vi "Send Throttle Signal.vi"(8 "error in (no error)":errorcluster, 9 "Requested Torque (Nm)":dbl format="%#_13g", 10 "CAN Offset":u32=160 format="%x", 11 "interface object in":refnum<k20>) -> (0 "error out":errorcluster, 3 "interface object out":refnum<k20>)   [LabVIEW 2014]
uses:
  <vilib>/RioEmbeddedCAN/RioEmbeddedCAN.llb/CANFrameControl.ctl
panel:
  in  "Direction":u8
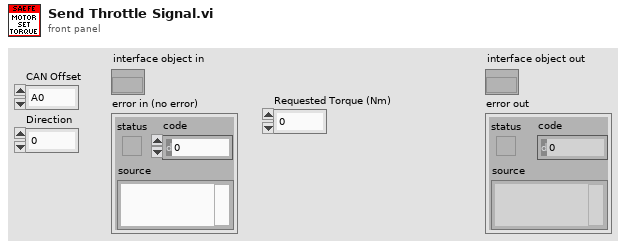
[diagram p1: front panel]
types:
  T1 = typedef "CANFrameControl.ctl" = cluster{"identifier":u32, "extended?":bool, "type":u8, "payload":u8[]}
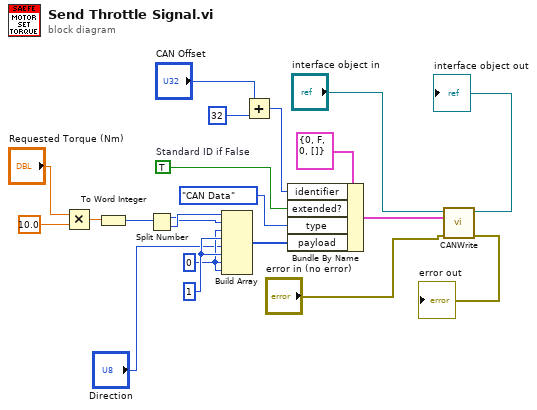
[diagram p0: block diagram]
diagram:
  w10 = u8 0 ("element")
  w11 = u8 1 ("element")
  w17 = TRUE  # Standard ID if False
  n1 = Multiply(x="Requested Torque (Nm)", y=10.0) -> (x*y=w4:dbl)
  n2 = To Word Integer(number=w4) -> (16bit integer=w3:i16)
  n3 = Split Number(x=w3) -> (hi(x)=w1:u8, lo(x)=w2:u8)
  n4 = Build Array(w2, w1, w10, w11, "Direction", w11, w10, w10) -> (w15:u8[])
  n5 = Add(x="CAN Offset", y=u32 32 ("identifier")) -> (x+y=w13:u32)
  n6 = Bundle By Name(cluster=T1 {"identifier"=0, "extended?"=FALSE, "type"=0, "payload"=[]} ("CAN frame"), "identifier"=w13, "extended?"=w17, "type"=enum8{"CAN Data", "CAN Remote"}."CAN Data", "payload"=w15) -> (w5:T1)
  n7 = call <vilib>:"CANWrite.vi"("error in (no error)"="error in (no error)", "CAN frame"=w5, "interface object in"="interface object in") -> ("error out"=→"error out":errorcluster, "interface object out"=→"interface object out":refnum<k20>)  [unwired: 7 in]
